vi "matlab_TI2_moveXY.vi"(8 "error in":errorcluster, 10 "deltaXY":cluster{dbl, dbl}) -> (0 "error out":errorcluster, 2 "XYZpos":cluster{dbl, dbl, dbl})   [LabVIEW 2018]
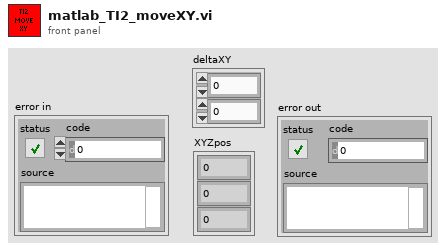
[diagram p1: front panel]
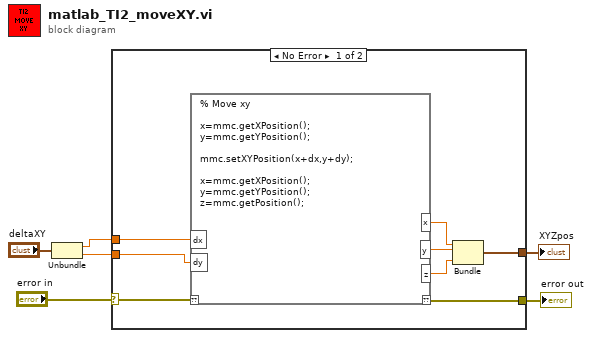
[diagram p0: block diagram]
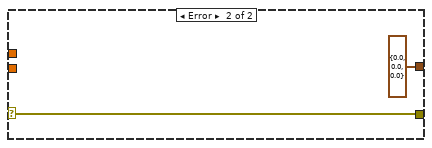
[diagram p2: hidden frame]
diagram:
  n1 = Unbundle("deltaXY") -> (w3:dbl, w2:dbl)
  n2 = case shown="No Error" "error in" {
    selector: "error in" -> [w14 w16]
    tunnel: [w13 w16] -> w5
    tunnel: w3 -> [w12 _]
    tunnel: w2 -> [w11 _]
    tunnel: [w7 cluster{dbl, dbl, dbl} {0.0, 0.0, 0.0}] -> w1
    frame No Error {
      n3 = script code="% Move xy\n\nx=mmc.getXPosition();\ny=mmc.getYPosition();\n\nmmc.setXYPosition(x+dx,y+dy);\n\nx=mmc.getXPosition();\ny=mmc.getYPosition();\nz=mmc.getPosition();"("??"=w14, "dx"=w12, "dy"=w11) -> ("??"=w13:errorcluster, "x"=w9:dbl, "y"=w10:dbl, "z"=w8:dbl)
      n4 = Bundle(w9, w10, w8) -> (w7:cluster{dbl, dbl, dbl})  [unwired: 1 in]
    }
    frame Error {
    }
  }
  "error out" <- w5
  "XYZpos" <- w1
